vi "Reactor Log.vi"(9 "Stop Chat":bool, 10 "Send":bool, 11 "Enter Text":string) -> (3 "Chat Window":string)   [LabVIEW 2017]
uses:
  <vilib>/OPCUA/controls/Write Status.ctl
  <vilib>/OPCUA/controls/NodeId.ctl
  <vilib>/OPCUA/client/Multiple Write String.vi
  <vilib>/OPCUA/NI OPC UA Client.lvlib
panel:
  out "Log Loop":i32
  out "Send Loop":i32
  in  "Node Status":T1 items=["Good"=0, "Uncertain_InitialValue"=1083310080, "Uncertain_LastUsableValue"=1083179008, "Uncertain_SensorNotAccurate"=1083375616, "Uncertain_EngineeringUnitsExceeded"=1083441152, "Bad_NoCommunication"=2150694912, "Bad_NotReadable"=2151284736, "Bad_NotWritable"=2151350272, "Bad_OutOfRange"=2151415808, "Bad_WaitingForInitialData"=2150760448]
  in  "Time Stamp":timestamp
  in  "Node Status":T1 items=["Good"=0, "Uncertain_InitialValue"=1083310080, "Uncertain_LastUsableValue"=1083179008, "Uncertain_SensorNotAccurate"=1083375616, "Uncertain_EngineeringUnitsExceeded"=1083441152, "Bad_NoCommunication"=2150694912, "Bad_NotReadable"=2151284736, "Bad_NotWritable"=2151350272, "Bad_OutOfRange"=2151415808, "Bad_WaitingForInitialData"=2150760448]
  in  "Time Stamp":timestamp
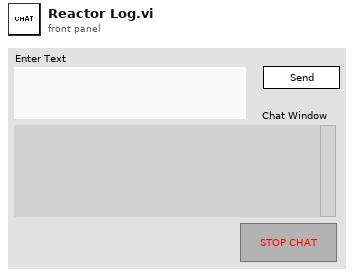
[diagram p1: front panel]
types:
  T1 = typedef "Write Status.ctl" = u32
  T2 = enum16{"open", "replace", "create", "open or create", "replace or create", "replace or create with confirmation"}
  T3 = typedef "OPC UA Client Refnum.ctl" = refnum<k21>
  T4 = typedef "NodeId.ctl" = string
  T5 = cluster{"node ID":T4, "value":string, "timestamp (current time)":timestamp, "node status":T1}
  T6 = cluster{"node ID":T4, "value":string, "timestamp (current time)":timestamp, "node status":T1}[]
  T7 = typedef "Subscription ID.ctl" = u32
  T8 = typedef "Subscription Data Change.ctl" = cluster{"node ID":T4, " value":variant, "timestamp":timestamp, "data type":T9, "status code":T10}
  T9 = typedef "Data Type.ctl" = u16
  T10 = typedef "OPC UA StatusCode.ctl" = u32
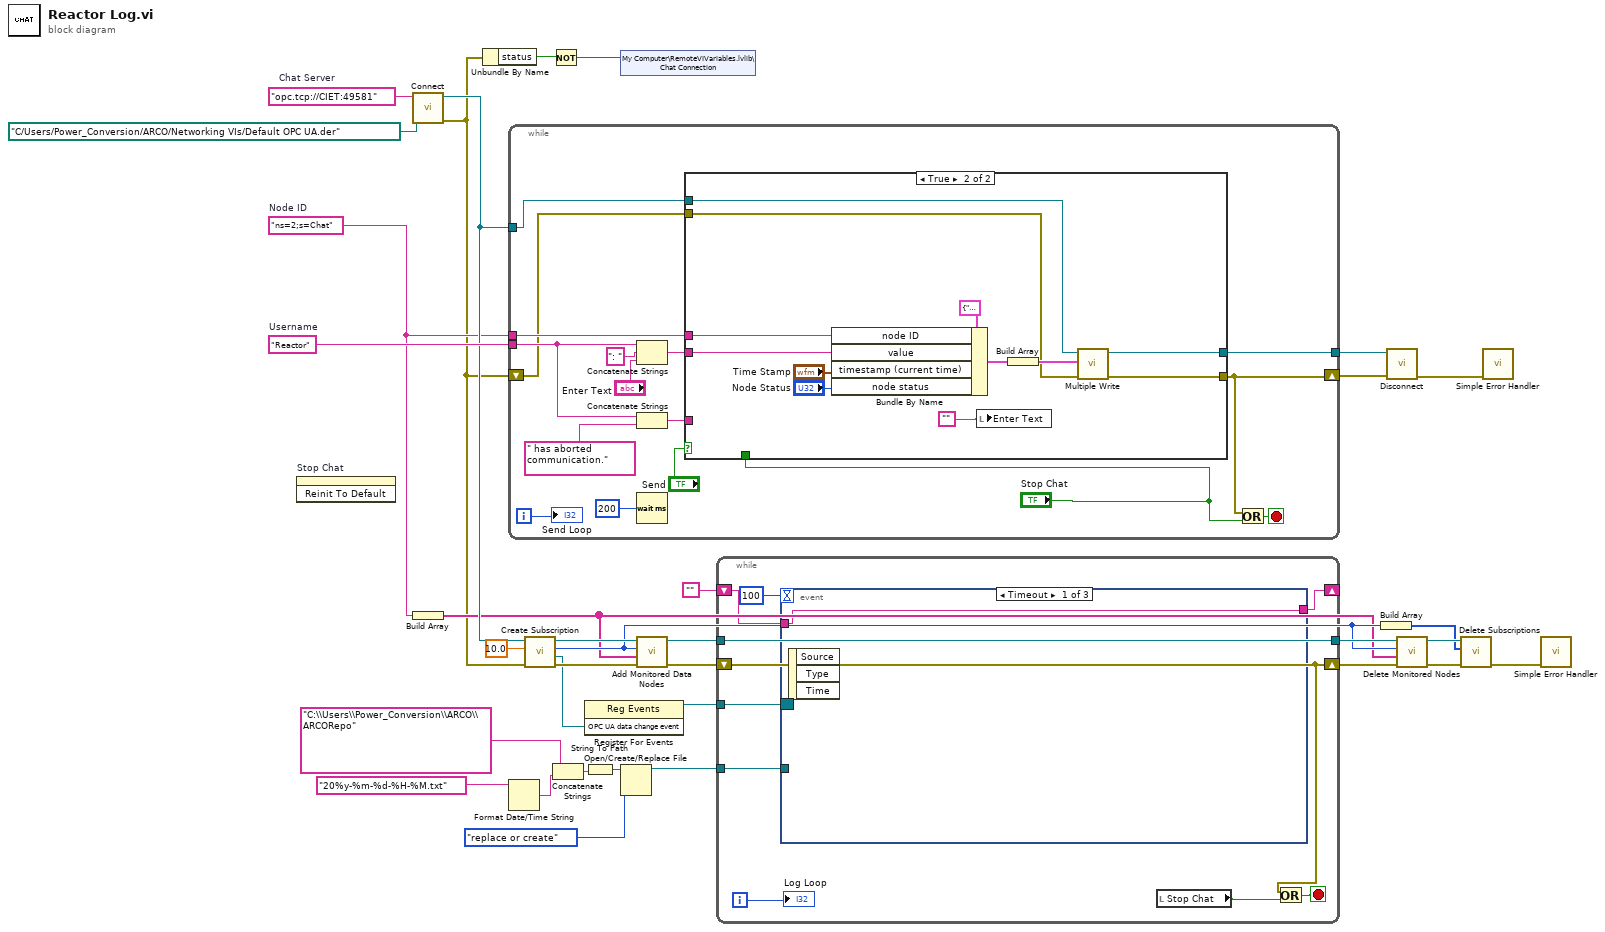
[diagram p0: block diagram]
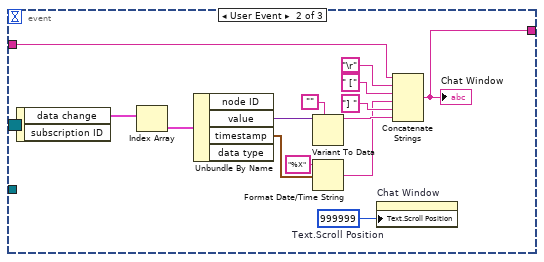
[diagram p2: hidden frame]
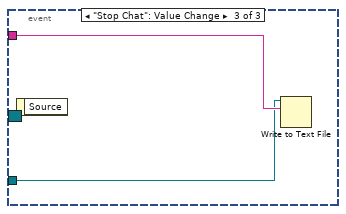
[diagram p3: hidden frame]
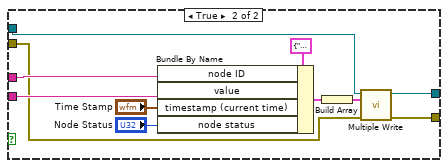
[diagram p5: hidden frame]
diagram:
  w16 = "ns=2;s=Chat"  # Node ID
  w32 = "Reactor"  # Username
  w33 = "opc.tcp://CIET:49581"  # Chat Server
  n1 = invoke on="Stop Chat" class="Bool (strict)" method="Reinit To Default"() -> ()  [unwired: 3 in, 3 out]
  n2 = call <vilib>:"Connect.vi"("client certificate file"=path "C:/Users/Power_Conversion/ARCO/Networking VIs/Default OPC UA.der", "server endpoint URL"=w33) -> ("error out"=w4:errorcluster, "OPC UA client refnum out"=w31:T3)  [unwired: 7 in, 1 out]
  n3 = Build Array(w16) -> (w15:string[])
  n4 = Unbundle By Name(w4) -> ("status"=w6:bool)
  n5 = while {
    tunnel: w16 -> [w42]
    tunnel: w32 -> [w47]
    tunnel: w31 -> [w40]
    tunnel: [w41] -> w13
    shift-right: [w35] -> w3
    shift-left: w4 -> [w39]
    i -> [w45]
    stop <- w37 stop-if-true
    n6 = Concatenate Strings(w47, ": ", "Enter Text") -> (w43:string)
    n7 = Concatenate Strings(w47, " has aborted communication.") -> (w38:string)
    n8 = Wait (ms)(milliseconds to wait=u32 200) -> ()  [unwired: 1 out]
    n9 = case shown="True" "Send" {
      tunnel: w43 -> [_ w77]
      tunnel: w42 -> [w55 w76]
      tunnel: [w51 w74] -> w41
      tunnel: [w52 w73] -> w35
      tunnel: w40 -> [w53 w72]
      tunnel: w39 -> [w54 w71]
      tunnel: "Stop Chat" -> [w57 _]
      tunnel: w38 -> [w56 _]
      frame False {
        n10 = case shown="False" w57 {
          tunnel: w56 -> [_ w65]
          tunnel: w55 -> [_ w64]
          tunnel: w54 -> [w58 w63]
          tunnel: w53 -> [w59 w62]
          tunnel: [w59 w61] -> w51
          tunnel: [w58 w60] -> w52
          frame False {
          }
          frame True {
            n11 = Bundle By Name(cluster=T5 {"node ID"="", "value"="", "timestamp (current time)"=timestamp(0 s since 1904-01-01), "node status"=0} ("request"), "node ID"=w64, "value"=w65, "timestamp (current time)"="Time Stamp", "node status"="Node Status") -> (w68:T5)
            n12 = Build Array(w68) -> (w67:T6)
            n13 = call-poly <vilib>:"Multiple Write.vi"("error in (no error)"=w63, "requests"=w67, "OPC UA client refnum in"=w62) -> ("error out"=w60:errorcluster, "OPC UA client refnum out"=w61:T3)  [unwired: 5 in, 2 out]
          }
        }
      }
      frame True {
        n14 = Bundle By Name(cluster=T5 {"node ID"="", "value"="", "timestamp (current time)"=timestamp(0 s since 1904-01-01), "node status"=0} ("request"), "node ID"=w76, "value"=w77, "timestamp (current time)"="Time Stamp", "node status"="Node Status") -> (w80:T5)
        n15 = local write "Enter Text"("") -> ()
        n16 = Build Array(w80) -> (w79:T6)
        n17 = call-poly <vilib>:"Multiple Write.vi"("error in (no error)"=w71, "requests"=w79, "OPC UA client refnum in"=w72) -> ("error out"=w73:errorcluster, "OPC UA client refnum out"=w74:T3)  [unwired: 5 in, 2 out]
      }
    }
    n18 = Or(x=w35, y="Stop Chat") -> (x .or. y?=w37:bool)
    "Send Loop" <- w45
  }
  n19 = Format Date/Time String(time format string (%c)="20%y-%m-%d-%H-%M.txt") -> (date/time string=w10:string)  [unwired: 2 in]
  n20 = call <vilib>:"Create Subscription.vi"("error in (no error)"=w4, "publishing interval (1000 ms)"=10.0, "OPC UA client refnum in"=w31) -> ("error out"=w29:errorcluster, "OPC UA data change event"=w28:refnum<user-event>, "subscription ID out"=w20:T7, "OPC UA client refnum out"=w30:T3)  [unwired: 4 in, 1 out]
  n21 = Not(x=w6) -> (.not. x?=w5:bool)
  n22 = Concatenate Strings("C:\\Users\\Power_Conversion\\ARCO\\ARCORepo", w10) -> (w8:string)
  n23 = register-events(w28) -> (reference out=w27:refnum<event-registration>)  [unwired: 2 in, 1 out]
  n24 = String To Path(string=w8) -> (path=w7:path)
  n25 = shared-variable "My Computer\\RemoteVIVariables.lvlib\\Chat Connection"(w5) -> ()  [unwired: 1 in, 1 out]
  n26 = Open/Create/Replace File(file path (use dialog)=w7, operation (0:open)=T2."replace or create") -> (refnum out=w17:refnum<file>)  [unwired: 4 in, 2 out]
  n27 = call <vilib>:"Add Monitored Data Nodes.vi"("error in (no error)"=w29, "node IDs"=w15, "subscription ID in"=w20, "OPC UA client refnum in"=w30) -> ("error out"=w23:errorcluster, "OPC UA client refnum out"=w25:T3)  [unwired: 4 in, 2 out]
  n28 = while {
    tunnel: w27 -> [w92]
    shift-right: [w90] -> _
    shift-left: "" -> [w91]
    tunnel: w25 -> [w89]
    tunnel: [w89] -> w24
    tunnel: w17 -> [w88]
    shift-right: [w84] -> w2
    shift-left: w23 -> [w84]
    i -> [w87]
    stop <- w85 stop-if-true
    n29 = event shown="[0] Timeout" {
      selector: w92 -> [_ _ _]
      dyn-events: _ -> [_ _ _]
      timeout: 100 -> [_ _ _]
      tunnel: w91 -> [w93 w96 w109]
      tunnel: [w93 w95 _] -> w90
      tunnel: w88 -> [_ _ w108]
      event Timeout {
        n30 = event-data() -> ()  [unwired: 1 in, 3 out]
      }
      event User Event {
        w94 = u32 999999  # Text.Scroll Position
        n31 = event-data() -> ("data change"=w107:T8[])  [unwired: 1 in, 1 out]
        n32 = Index Array(array=w107) -> (element=w106:T8)  [unwired: 1 in]
        n33 = Unbundle By Name(w106) -> ("value"=w105:variant, "timestamp"=w103:timestamp)  [unwired: 2 out]
        n34 = Variant To Data(type="", Variant=w105) -> (data=w101:string)  [unwired: 1 in, 1 out]
        n35 = Format Date/Time String(time format string (%c)="%X", seconds (now)=w103) -> (date/time string=w99:string)  [unwired: 1 in]
        n36 = property on="Chat Window" class="Str"("Text.Scroll Position"=w94) -> ()  [unwired: 2 in, 2 out]
        n37 = Concatenate Strings(w96, "\r", " [", w99, "] ", w101) -> (w95:string)
        "Chat Window" <- w95
      }
      event "Stop Chat": Value Change {
        n38 = event-data() -> ()  [unwired: 1 in, 1 out]
        n39 = Write to Text File(file (use dialog)=w108, text=w109) -> ()  [unwired: 2 in, 3 out]
      }
    }
    n40 = local read "Stop Chat"() -> (w83:bool)
    n41 = Or(x=w84, y=w83) -> (x .or. y?=w85:bool)
    "Log Loop" <- w87
  }
  n42 = Build Array(w20) -> (w19:T7[])
  n43 = call <vilib>:"Disconnect.vi"("error in (no error)"=w3, "OPC UA client refnum in"=w13) -> ("error out"=w34:errorcluster)  [unwired: 9 in]
  n44 = call <vilib>:"Delete Monitored Nodes.vi"("error in (no error)"=w2, "node IDs"=w15, "subscription ID in"=w20, "OPC UA client refnum in"=w24) -> ("error out"=w21:errorcluster, "OPC UA client refnum out"=w22:T3)  [unwired: 3 in, 3 out]
  n45 = call <vilib>:"Delete Subscriptions.vi"("error in (no error)"=w21, "subscription IDs"=w19, "OPC UA client refnum in"=w22) -> ("error out"=w18:errorcluster)  [unwired: 6 in, 2 out]
  n46 = call <vilib>:"Simple Error Handler.vi"("error in (no error)"=w34) -> ()  [unwired: 4 in, 5 out]
  n47 = call <vilib>:"Simple Error Handler.vi"("error in (no error)"=w18) -> ()  [unwired: 4 in, 5 out]
